vi "Launcher.vi"() -> ()   [LabVIEW 2020]
uses:
  UI Actor.lvclass
  C:/Program Files (x86)/National Instruments/LabVIEW 2020/vi.lib/ActorFramework/Actor/Actor.lvclass
  Impemetnations/NXP/NXP.lvclass
  Impemetnations/Arduino/Arduino.lvclass
  Impemetnations/Simulado/Simulado.lvclass
  UI Actor.lvclass/UI Actor.ctl
  Write VISA resource name.vi
  Write Serial Device.lvclass.vi
  <vilib>/Instr/_visa.llb/VISA Configure Serial Port (Instr).vi
  <vilib>/ActorFramework/Actor/Actor.lvclass
panel:
  in  "Microcontroller":enum16{"NXP", "Arduino", "Simulated"}(ring)
  in  "COM Port":refnum<visa-resource-name>
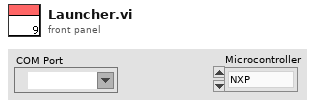
[diagram p1: front panel]
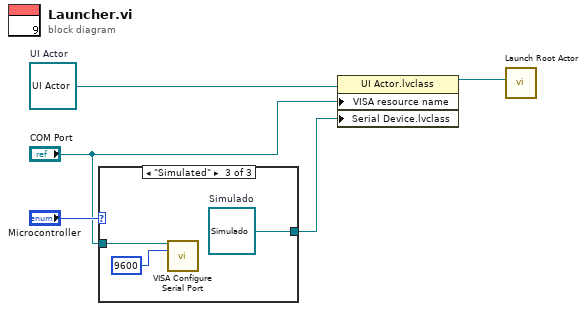
[diagram p0: block diagram]
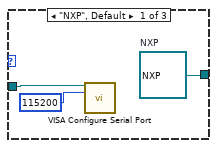
[diagram p2: hidden frame]
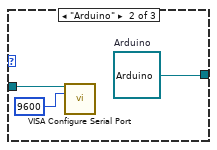
[diagram p3: hidden frame]
diagram:
  w5 = refnum<class "UI Actor.lvclass"> refnum  # UI Actor
  n1 = case shown="\"Simulated\"" "Microcontroller" {
    tunnel: [w8 w11 w14] -> w2
    tunnel: "COM Port" -> [w7 w10 w13]
    frame "NXP", Default {
      w8 = refnum<class "NXP.lvclass"> refnum  # NXP
      n2 = call-poly "VISA Configure Serial Port"("VISA resource name"=w7, "baud rate (9600)"=u32 115200) -> ()  [unwired: 12 in, 2 out]
    }
    frame "Arduino" {
      w11 = refnum<class "Arduino.lvclass"> refnum  # Arduino
      n3 = call-poly "VISA Configure Serial Port"("VISA resource name"=w10, "baud rate (9600)"=u32 9600) -> ()  [unwired: 12 in, 2 out]
    }
    frame "Simulated" {
      w14 = refnum<class "Simulado.lvclass"> refnum  # Simulado
      n4 = call-poly "VISA Configure Serial Port"("VISA resource name"=w13, "baud rate (9600)"=u32 9600) -> ()  [unwired: 12 in, 2 out]
    }
  }
  n5 = property class="UI Actor.lvclass"(reference=w5, "VISA resource name"="COM Port", "Serial Device.lvclass"=w2) -> (reference out=w4:refnum<class "UI Actor.lvclass">)  [unwired: 1 in, 1 out]
  n6 = call <vilib>:"Launch Root Actor.vi"("Actor"=w4) -> ()  [unwired: 9 in, 2 out]
